vi "App enquece.vi"(6 "Priority Enquece":bool, 8 "error in (no error)":errorcluster, 9 "command data":variant, 10 "command":string="INIT.Read HW config", 11 "queue in":refnum<queue>) -> (0 "error out":errorcluster, 3 "Queue out":refnum<queue>)   [LabVIEW 2018, in "Application.lvlib"]
uses:
  Application.lvlib
  App state data.ctl
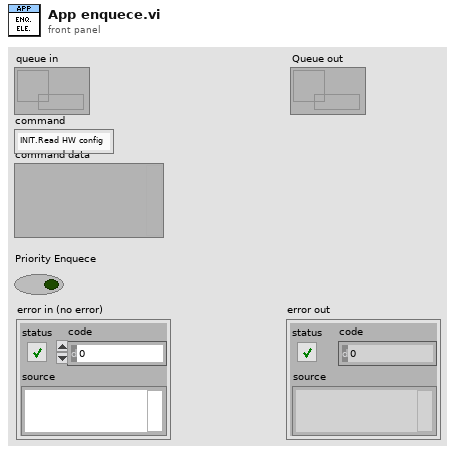
[diagram p1: front panel]
types:
  T1 = typedef "Application.lvlib/App state data.ctl" = cluster{"command":string, "command data":variant}
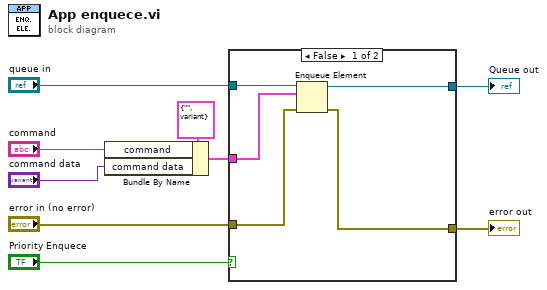
[diagram p0: block diagram]
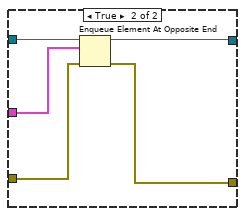
[diagram p2: hidden frame]
diagram:
  n1 = Bundle By Name(cluster=T1 {"command"="", "command data"=variant} ("element"), "command"="command", "command data"="command data") -> (w9:T1)
  n2 = case shown="False" "Priority Enquece" {
    tunnel: w9 -> [w10 w17]
    tunnel: "queue in" -> [w14 w19]
    tunnel: "error in (no error)" -> [w13 w16]
    tunnel: [w12 w15] -> w5
    tunnel: [w11 w18] -> w4
    frame False {
      n3 = Enqueue Element(queue=w14, element=w10, error in (no error)=w13) -> (queue out=w11:refnum<queue>, error out=w12:errorcluster)  [unwired: 1 in, 1 out]
    }
    frame True {
      n4 = Enqueue Element At Opposite End(queue=w19, element=w17, error in (no error)=w16) -> (queue out=w18:refnum<queue>, error out=w15:errorcluster)  [unwired: 1 in, 1 out]
    }
  }
  "error out" <- w5
  "Queue out" <- w4
